vi "Check IDs in XML.vi"(8 "Error In":errorcluster, 11 "XML Path":path) -> (0 "Error Out":errorcluster)   [LabVIEW 2019, in "Tools.lvlib"]
uses:
  Tools.lvlib
  <vilib>/xml/Load XML File.vi
  <vilib>/xml/Close Reference(Node).vi
  <vilib>/xml/NI_XML.lvlib
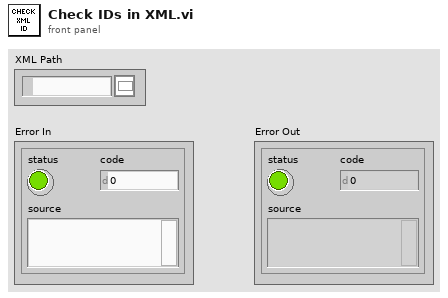
[diagram p1: front panel]
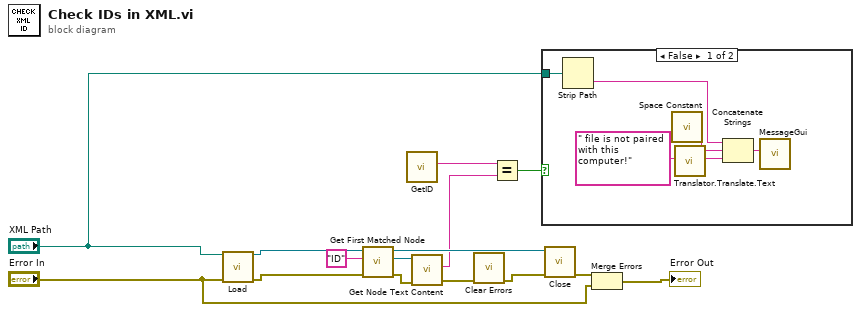
[diagram p0: block diagram]
diagram:
  n1 = call-poly <vilib>:"Load.vi"("path to XML document"="XML Path", "error in (no error)"="Error In") -> ("DOM document out"=w10:refnum<k20>, "error out"=w12:errorcluster)  [unwired: 11 in, 1 out]
  n2 = call <vilib>:"Get First Matched Node.vi"("error in (no error)"=w12, "XPath expression"="ID", "node in"=w10) -> ("error out"=w13:errorcluster, "node result"=w14:refnum<k20>, "node out"=w11:refnum<k20>)  [unwired: 6 in]
  n3 = call "GetID.vi"() -> ("Computer ID"=w9:string)  [unwired: 10 in, 1 out]
  n4 = call <vilib>:"Get Node Text Content.vi"("error in (no error)"=w13, "node in"=w14) -> ("error out"=w7:errorcluster, "node text"=w8:string)  [unwired: 7 in, 1 out]
  n5 = call <vilib>:"Clear Errors.vi"("error in (no error)"=w7) -> ("error out"=w6:errorcluster)  [unwired: 5 in, 1 out]
  n6 = Equal?(x=w9, y=w8) -> (x = y?=w2:bool)
  n7 = case shown="False" w2 {
    tunnel: "XML Path" -> [w21 _]
    frame False {
      n8 = Strip Path(path=w21) -> (name=w19:string)  [unwired: 1 out]
      n9 = call <vilib>:"Space Constant.vi"() -> ("String"=w20:string)
      n10 = call "Translator.Translate.Text.vi"("text"=" file is not paired with this computer!") -> ("translated text"=w17:string)  [unwired: 9 in, 1 out]
      n11 = Concatenate Strings(w19, w20, w17) -> (w16:string)
      n12 = call "MessageGui.vi"("Message"=w16) -> ()  [unwired: 10 in, 1 out]
    }
    frame True {
    }
  }
  n13 = call-poly <vilib>:"Close.vi"("error in (no error)"=w6, "node"=w11) -> ("error out"=w5:errorcluster)  [unwired: 7 in]
  n14 = Merge Errors(w5, "Error In") -> (→"Error Out":errorcluster)
